vi "Sizeof.Array.vi"(10 "count":i32, 11 "data type":T1) -> (3 "size":i32)   [LabVIEW 2016, in "VeriStand Data.lvlib"]
doc: "Provides the size in bytes of an array of length <B>count</B> for a specified <B>data type</B>."
uses:
  VeriStand Data.lvlib
  Typedefs/Typedefs.Data Types.ctl
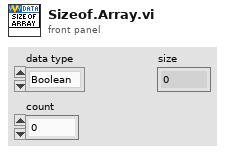
[diagram p1: front panel]
types:
  T1 = typedef "VeriStand Data.lvlib/Typedefs.Data Types.ctl" = enum16{"Boolean", "Single", "Double", "I8", "I16", "I32", "I64", "U8", "U16", "U32", "U64"}
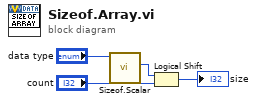
[diagram p0: block diagram]
diagram:
  n1 = call "Sizeof.Scalar.vi"("data type"="data type") -> ("bitshift count"=w2:u8)  [unwired: 9 in, 1 out]
  n2 = Logical Shift(y=w2, x="count") -> (x << y=→"size":i32)
